vi "Registers.Initialize.vi"(7 "Group.Rate":u32[](array[numeric]), 8 "error in (no error)":errorcluster, 9 "Values":dbl[](array[numeric]), 10 "Registers":T1[](array[typedef]) {"Register"."Data Type" format="%.0x"}, 11 "FPGA Ref":refnum<k20>) -> (0 "error out":errorcluster, 2 "Registers Ref":T4[](array[typedef]) {"Data Type" format="%.0x"}, 3 "FPGA Ref out":refnum<k20>)   [LabVIEW 2019, in "Fuel Injector Analysis Addon Engine.lvlib"]
uses:
  Fuel Injector Analysis Addon Engine.lvlib
  Types/FPGA Refs.ctl
  Addon Shared/Types/FPGA Data Types.ctl
  Addon Shared/Types/VS.Register.Info.ctl
  Addon Shared/Types/Register.Info.ctl
  Addon Shared/Fuel Injector Analysis Addon Shared.lvlib
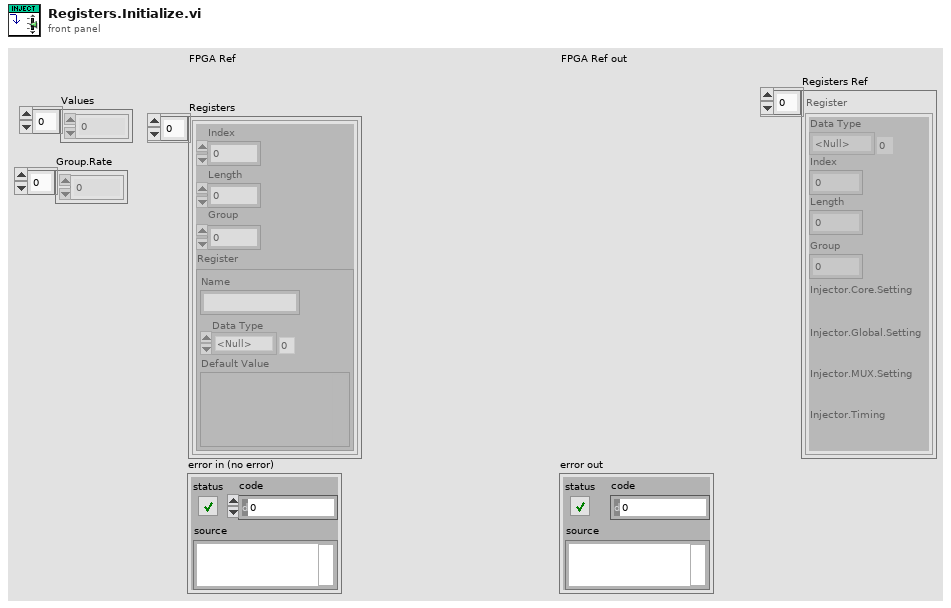
[diagram p1: front panel]
types:
  T1 = typedef "Fuel Injector Analysis Addon Shared.lvlib/VS.Register.Info.ctl" = cluster{"Index":i32, "Length":i32, "Group":i32, "Register":T2}
  T2 = typedef "Fuel Injector Analysis Addon Shared.lvlib/Register.Info.ctl" = cluster{"Name":string, "Data Type":T3, "Default Value":variant}
  T3 = typedef "Fuel Injector Analysis Addon Shared.lvlib/FPGA Data Types.ctl" = enum8{"<Null>", "Injector.Core.Setting", "Injector.Global.Setting", "Injector.Mux.Setting", "Injector.Timing"}
  T4 = typedef "Fuel Injector Analysis Addon Engine.lvlib/FPGA Refs.ctl" = cluster{"Data Type":T3, "Index":i32, "Length":i32, "Group":i32, "Injector.Core.Setting":refnum<k20>, "Injector.Global.Setting":refnum<k20>, "Injector.MUX.Setting":refnum<k20>, "Injector.Timing":refnum<k20>}
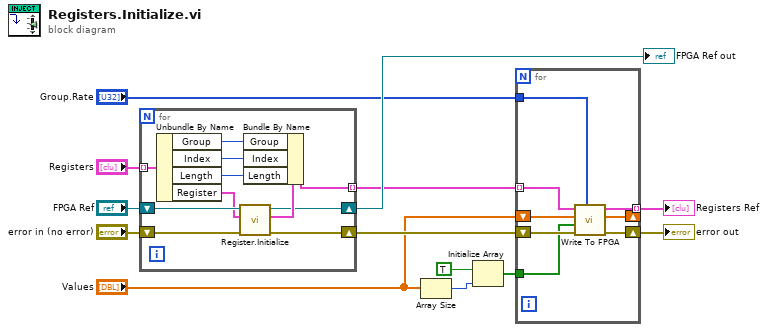
[diagram p0: block diagram]
diagram:
  n1 = for {
    shift-right: [w15] -> w5
    shift-left: "FPGA Ref" -> [w20]
    tunnel: [w24] -> w4 mode=indexing
    tunnel: "Registers" -> [w23] mode=indexing
    shift-right: [w16] -> w9
    shift-left: "error in (no error)" -> [w19]
    n2 = Unbundle By Name(w23) -> ("Group"=w14:i32, "Index"=w21:i32, "Length"=w22:i32, "Register"=w17:T2)
    n3 = call "Register.Initialize.vi"("error in (no error)"=w19, "Register"=w17, "FPGA Ref"=w20) -> ("error out"=w16:errorcluster, "Register out"=w18:T4, "FPGA Ref out"=w15:refnum<k20>)  [unwired: 6 in]
    n4 = Bundle By Name(cluster=w18, "Group"=w14, "Index"=w21, "Length"=w22) -> (w24:T4)
  }
  "FPGA Ref out" <- w5
  n5 = Array Size(array="Values") -> (size(s)=w8:i32)
  n6 = Initialize Array(TRUE, w8) -> (w6:bool[])
  n7 = for {
    shift-right: [w28] -> _
    shift-left: "Values" -> [w29]
    shift-right: [w31] -> w10
    shift-left: w9 -> [w32]
    tunnel: w6 -> [w30]
    tunnel: "Group.Rate" -> [w27]
    tunnel: w4 -> [w26] mode=indexing
    tunnel: [w25] -> w3 mode=indexing
    n8 = call "Write To FPGA.vi"("Group.Rate"=w27, "error in (no error)"=w32, "Changed?"=w30, "Values"=w29, "FPGA Refs"=w26) -> ("error out"=w31:errorcluster, "Values out"=w28:dbl[], "FPGA Refs"=w25:T4)  [unwired: 4 in]
  }
  "error out" <- w10
  "Registers Ref" <- w3
